vi "xyCoordinateTransform.vi"(0 "Point in":cluster{dbl, dbl}, 3 "Transform (Center first)":T1={"Center"={0.0, 0.0}, "Rotate (rad)"=0.0, "MirrorY"=FALSE, "Scale"=1.0}, 4 "Back":bool) -> (2 "Point Out":cluster{dbl, dbl})   [LabVIEW 2011]
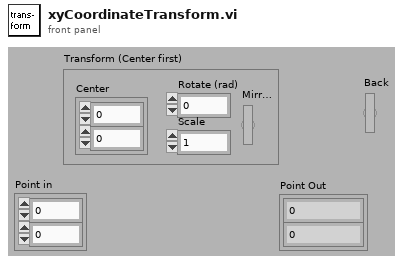
[diagram p1: front panel]
types:
  T1 = cluster{"Center":cluster{dbl, dbl}, "Rotate (rad)":dbl, "MirrorY":bool, "Scale":dbl}
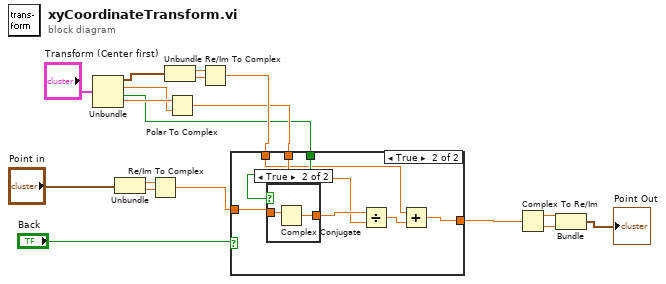
[diagram p0: block diagram]
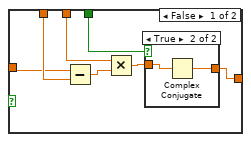
[diagram p2: hidden frame]
diagram:
  n1 = Unbundle("Transform (Center first)") -> ("Center"=w15:cluster{dbl, dbl}, "Rotate (rad)"=w12:dbl, "MirrorY"=w10:bool, "Scale"=w13:dbl)
  n2 = Unbundle("Point in") -> (w6:dbl, w5:dbl)
  n3 = Re/Im To Complex(1:w5, 2:w6) -> (0:w4:cdb)
  n4 = Unbundle(w15) -> (w17:dbl, w16:dbl)
  n5 = Polar To Complex(1:w12, 2:w13) -> (0:w11:cdb)
  n6 = Re/Im To Complex(1:w16, 2:w17) -> (0:w14:cdb)
  n7 = case shown="True" "Back" {
    tunnel: w14 -> [w24 w31]
    tunnel: w11 -> [w23 w32]
    tunnel: w10 -> [w21 w34]
    tunnel: w4 -> [w20 w30]
    tunnel: [w19 w29] -> w1
    frame False {
      n8 = Subtract(x=w20, y=w24) -> (x-y=w25:cdb)
      n9 = Multiply(x=w23, y=w25) -> (x*y=w22:cdb)
      n10 = case shown="True" w21 {
        tunnel: w22 -> [w26 w28]
        tunnel: [w26 w27] -> w19
        frame False {
        }
        frame True {
          n11 = Complex Conjugate(1:w28) -> (0:w27:cdb)
        }
      }
    }
    frame True {
      n12 = case shown="True" w34 {
        tunnel: [w36 w38] -> w35
        tunnel: w30 -> [w36 w37]
        frame False {
        }
        frame True {
          n13 = Complex Conjugate(1:w37) -> (0:w38:cdb)
        }
      }
      n14 = Divide(x=w35, y=w32) -> (x/y=w33:cdb)
      n15 = Add(x=w31, y=w33) -> (x+y=w29:cdb)
    }
  }
  n16 = Complex To Re/Im(x + iy=w1) -> (x=w3:dbl, y=w2:dbl)
  n17 = Bundle(w3, w2) -> (→"Point Out":cluster{dbl, dbl})  [unwired: 1 out]
